vi "15-2.vi"() -> ()   [LabVIEW 2019, in "15.lvlib"]
uses:
  15.lvlib
panel:
  in  "Sample Input?":bool
  out "Lowest Risk":u64
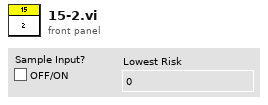
[diagram p1: front panel]
types:
  T1 = map{cluster{"Row":i32, "Col":i32}, cluster{"Adjacency Matrix":cluster{i32, i32}[], "Risk":u8, "Min Risk":i32, "Visited?":bool}}
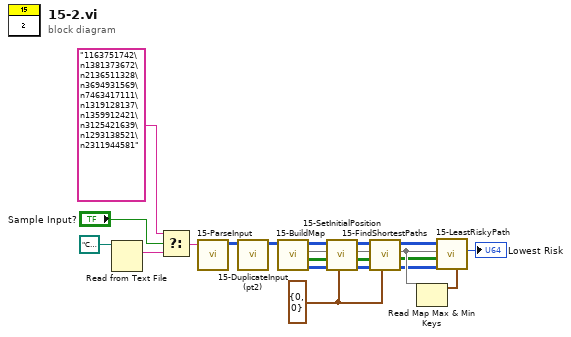
[diagram p0: block diagram]
diagram:
  w2 = cluster{"Row":i32, "Col":i32} {"Row"=0, "Col"=0} ("Initial Position in")
  n1 = Read from Text File(file (use dialog)=path "C:/Users/craig.walker/Documents/GitHub/lv2019-Advent-of-Code-2021/15/input.txt") -> (text=w16:string)  [unwired: 3 in, 3 out]
  n2 = Select(t="1163751742\n1381373672\n2136511328\n3694931569\n7463417111\n1319128137\n1359912421\n3125421639\n1293138521\n2311944581", s="Sample Input?", f=w16) -> (s? t:f=w17:string)
  n3 = call "15-ParseInput.vi"("String"=w17) -> ("Risk Array"=w18:u8[][])  [unwired: 10 in]
  n4 = call "15-DuplicateInput(pt2).vi"("Risk Array in"=w18) -> ("Risk Array out"=w7:u8[][])  [unwired: 10 in]
  n5 = call "15-BuildMap.vi"("Risk Array in"=w7) -> ("Min Risk Array"=w6:i32[][], "Visited Array"=w9:bool[][], "map"=w19:T1, "Risk Array out"=w21:u8[][])  [unwired: 7 in]
  n6 = call "15-SetInitialPosition.vi"("Initial Position in"=w2, "Min Risk Array in"=w6, "Visited Array in"=w9, "map in"=w19, "Risk Array in"=w21) -> ("Min Risk Array out"=w10:i32[][], "Visited Array out"=w8:bool[][], "map out"=w13:T1, "Risk Array out"=w20:u8[][])  [unwired: 3 in]
  n7 = call "15-FindShortestPaths.vi"("Initial Position in"=w2, "Min Risk Array in"=w10, "Visited Array in"=w8, "map in"=w13, "Risk Array in"=w20) -> ("Min Risk Array out"=w4:i32[][], "Visited Array out"=w3:bool[][], "map out"=w11:T1, "Risk Array out"=w5:u8[][])  [unwired: 3 in]
  n8 = Read Map Max & Min Keys(11:w11) -> (3:w1:cluster{"Row":i32, "Col":i32})  [unwired: 1 out]
  n9 = call "15-LeastRiskyPath.vi"("Final Position"=w1, "Min Risk Array in"=w4, "Visited Array in"=w3, "map in"=w11, "Risk Array in"=w5) -> ("Min Risk"=→"Lowest Risk":i32)  [unwired: 3 in, 3 out]
